vi "Paths.vi"() -> (3 "Paths":T1)   [LabVIEW 2022 SP3, in "FlexBlocks Support.lvlib"]
uses:
  FlexBlocks Support.lvlib
  Paths.ctl
  <vilib>/Utility/sysdir.llb/System Directory Type.ctl
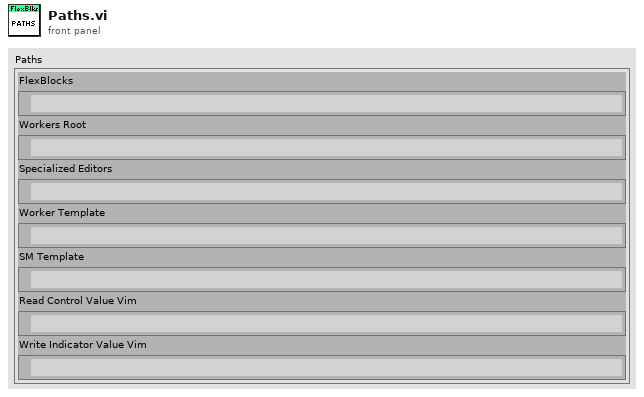
[diagram p1: front panel]
types:
  T1 = typedef "FlexBlocks Support.lvlib/Paths.ctl" = cluster{"FlexBlocks":path, "Workers Root":path, "Specialized Editors":path, "Worker Template":path, "SM Template":path, "Read Control Value Vim":path, "Write Indicator Value Vim":path}
  T2 = typedef "System Directory Type.ctl" = i32
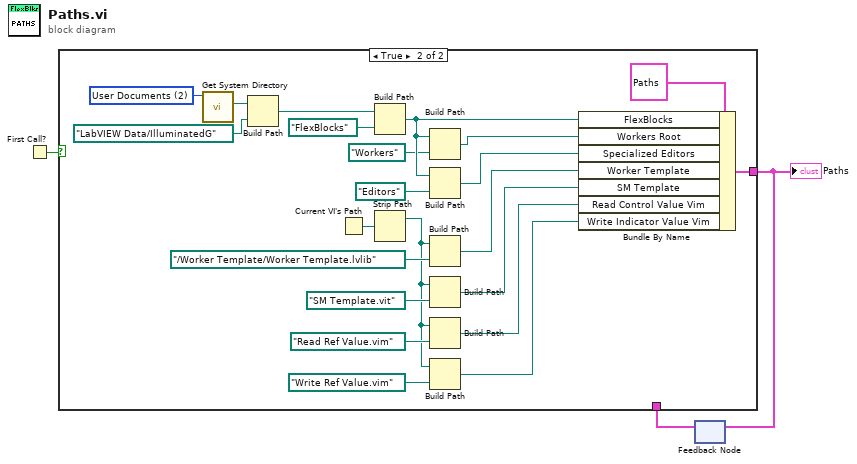
[diagram p0: block diagram]
diagram:
  n1 = First Call?() -> (First Call?: T/F=w3:bool)
  n2 = feedback #1() -> (w1:T1)  [unwired: 1 in]
  n3 = case shown="True" w3 {
    tunnel: [w4 w20] -> w2
    tunnel: w1 -> [w4 _]
    frame False {
    }
    frame True {
      w8 = T2 2 items=["User Home"=0, "User Desktop"=1, "User Documents"=2, "User Application Data"=3, "User Preferences"=4, "User Temporary"=5, "Public Documents"=6, "Public Application Data"=7, "Public Preferences"=8, "Public Cache"=13, "System Core Libraries"=9, "System Installed Libraries"=10, "Application Files"=11, "Boot Volume Root"=12] ("system directory type")
      n4 = call <vilib>:"Get System Directory.vi"("system directory type"=w8) -> ("system directory"=w7:path)  [unwired: 10 in]
      n5 = Build Path(base path=w7, name or relative path=path "LabVIEW Data/IlluminatedG") -> (appended path=w5:path)
      n6 = Current VI's Path() -> (path=w19:path)
      n7 = Build Path(base path=w5, name or relative path=path "FlexBlocks") -> (appended path=w25:path)
      n8 = Strip Path(path=w19) -> (stripped path=w10:path)  [unwired: 1 out]
      n9 = Build Path(base path=w25, name or relative path=path "Workers") -> (appended path=w23:path)
      n10 = Build Path(base path=w25, name or relative path=path "Editors") -> (appended path=w21:path)
      n11 = Build Path(base path=w10, name or relative path=path "../Worker Template/Worker Template.lvlib") -> (appended path=w16:path)
      n12 = Build Path(base path=w10, name or relative path=path "SM Template.vit") -> (appended path=w13:path)
      n13 = Build Path(base path=w10, name or relative path=path "Read Ref Value.vim") -> (appended path=w12:path)
      n14 = Build Path(base path=w10, name or relative path=path "Write Ref Value.vim") -> (appended path=w9:path)
      n15 = Bundle By Name(cluster=T1 {"FlexBlocks"=path "", "Workers Root"=path "", "Specialized Editors"=path "", "Worker Template"=path "", "SM Template"=path "", "Read Control Value Vim"=path "", "Write Indicator Value Vim"=path ""} ("Paths"), "FlexBlocks"=w25, "Workers Root"=w23, "Specialized Editors"=w21, "Worker Template"=w16, "SM Template"=w13, "Read Control Value Vim"=w12, "Write Indicator Value Vim"=w9) -> (w20:T1)
    }
  }
  "Paths" <- w2
  n16 = feedback-in #1(w2) -> ()
